vi "factorial.vi"() -> ()   [LabVIEW 2017]
panel:
  out "factorial":dbl
  in  "Numeric":dbl
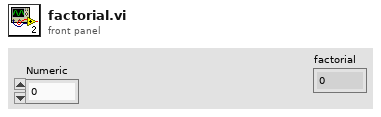
[diagram p1: front panel]
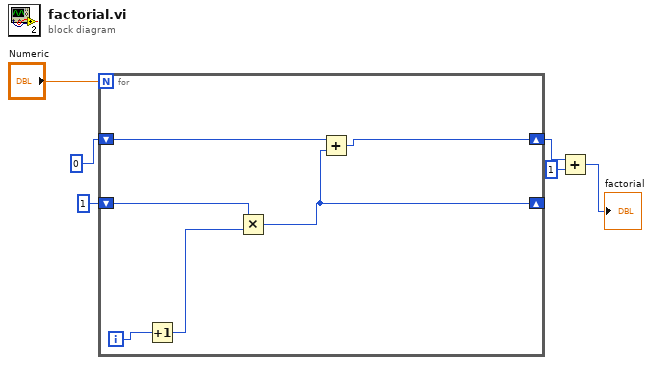
[diagram p0: block diagram]
diagram:
  n1 = for {
    N: "Numeric" -> [_]
    shift-right: [w7] -> _
    shift-left: 1 -> [w10]
    shift-right: [w9] -> w3
    shift-left: 0 -> [w8]
    i -> [w12]
    n2 = Increment(x=w12) -> (x+1=w11:i32)
    n3 = Multiply(x=w10, y=w11) -> (x*y=w7:i32)
    n4 = Add(x=w8, y=w7) -> (x+y=w9:i32)
  }
  n5 = Add(x=w3, y=1) -> (x+y=→"factorial":i32)
